vi "Launcher.vi"   [LabVIEW 2020]
uses:
  gui/gui.lvclass
  C:/Program Files (x86)/National Instruments/LabVIEW 2020/vi.lib/ActorFramework/Actor/Actor.lvclass
  <vilib>/ActorFramework/Actor/Actor.lvclass
panel:
  # "Just Launcher"
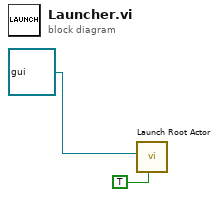
[diagram p0: block diagram]
diagram:
  n1 = call <vilib>:"Launch Root Actor.vi"("Open Actor Core front panel? (F)"=TRUE, "Actor"=refnum<class "gui.lvclass"> refnum ("gui.lvlib:gui.lvclass")) -> ()  [unwired: 8 in, 2 out]
